vi "Get SSL Stream.vi"(6 "Leave Inner Stream Open":bool, 8 "Error In":errorcluster, 11 "Client Ref":refnum<k24>) -> (0 "Error Out":errorcluster, 2 "SSL Ref":refnum<k24>, 3 "Client Ref":refnum<k24>)   [LabVIEW 2014, in "SSL Lib.lvlib"]
doc: "VI Function: This VI gives SSL stream reference after a client is connected.\n\nVI Version: 1.0\n\nVI Author: Runjhun Agarwal"
uses:
  <userlib>/SSL Library/SSL Lib.lvlib
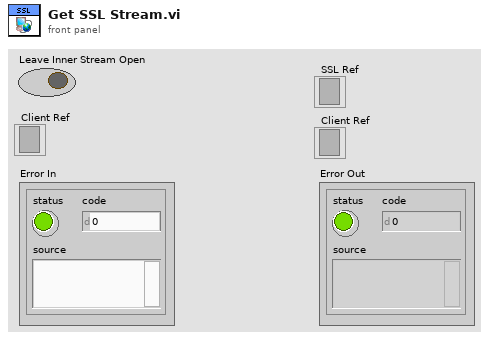
[diagram p1: front panel]
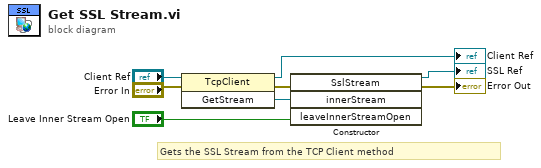
[diagram p0: block diagram]
diagram:
  # "Gets the SSL Stream from the TCP Client method"
  n1 = invoke class="TcpClient" method="GetStream"(reference="Client Ref", error in="Error In") -> (reference out=→"Client Ref":refnum<k24>, error out=w4:errorcluster, "GetStream"=w7:refnum<k24>)  [unwired: 1 in]
  n2 = constructor class="SslStream"(error in=w4, "innerStream"=w7, "leaveInnerStreamOpen"="Leave Inner Stream Open") -> (reference out=→"SSL Ref":refnum<k24>, error out=→"Error Out":errorcluster)  [unwired: 2 in, 3 out]
